vi "PythagFindH.vi"(1 "Side B":dbl, 2 "Side A":dbl) -> (0 "Side H":dbl)   [LabVIEW 2016]
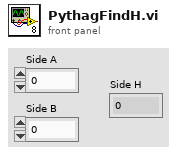
[diagram p1: front panel]
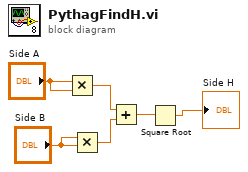
[diagram p0: block diagram]
diagram:
  n1 = Multiply(x="Side A", y="Side A") -> (x*y=w6:dbl)
  n2 = Multiply(x="Side B", y="Side B") -> (x*y=w5:dbl)
  n3 = Add(x=w6, y=w5) -> (x+y=w4:dbl)
  n4 = Square Root(x=w4) -> (sqrt(x)=→"Side H":dbl)
